vi "Read File Attributes.vi"(8 "error in (no error)":errorcluster, 10 "File (\"D:\\user\\data\")":string="D:\\user\\data", 11 "VISA resource name":refnum<visa-resource-name>) -> (0 "error out":errorcluster, 2 "Output":string, 3 "VISA resource name out":refnum<visa-resource-name>)   [LabVIEW 2015, in "Rohde&Schwarz CMXP Base.lvlib"]
doc: "Reads file properties for files and directories.\n\nAttribute:\n-\n\nRemote-control command:\nMMEMory:ATTRibute?"
uses:
  <instrlib>/Rohde&Schwarz CMXP Base/Rohde&Schwarz CMXP Base.lvlib
  <instrlib>/Rohde&Schwarz CMXP Base/Private/rsidr_core.llb/rsidr_core.lvlib
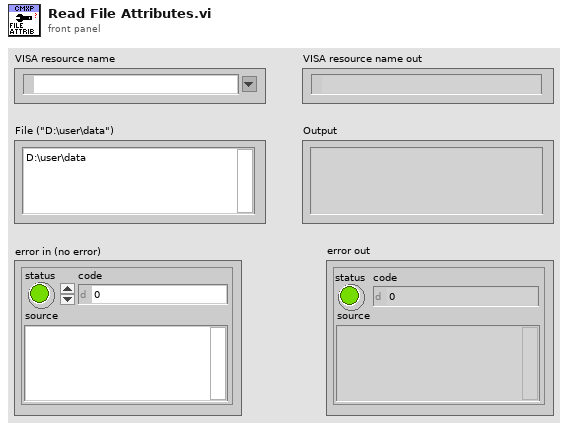
[diagram p1: front panel]
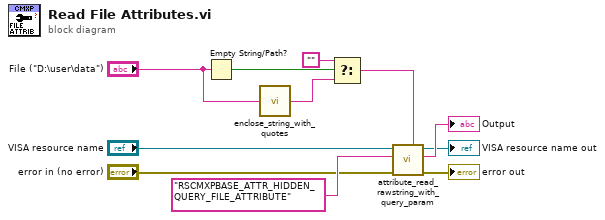
[diagram p0: block diagram]
diagram:
  n1 = Empty String/Path?(string/path="File (\"D:\\user\\data\")") -> (empty?=w4:bool)
  n2 = call <instrlib>:"enclose_string_with_quotes.vi"("String to enclose"="File (\"D:\\user\\data\")") -> ("String out"=w1:string)  [unwired: 4 in]
  n3 = Select(t="" ("Empty String Constant"), s=w4, f=w1) -> (s? t:f=w3:string)
  n4 = call <instrlib>:"attribute_read_rawstring_with_query_param.vi"("Query Parameter (None)"=w3, "error in"="error in (no error)", "Attribute ID"="RSCMXPBASE_ATTR_HIDDEN_QUERY_FILE_ATTRIBUTE", "VISA resource name"="VISA resource name") -> ("error out"=→"error out":errorcluster, "RawString out"=→"Output":string, "VISA resource name out"=→"VISA resource name out":refnum<visa-resource-name>)  [unwired: 5 in]
